vi "LeCroy Wave Series Acquire Waveform.vi"() -> ()   [LabVIEW 2015]
doc: "This example shows how to use autosetup and acquire a waveform on a single channel."
uses:
  Public/Data/Read Single Waveform.vi
  LeCroy Wave Series.lvlib
panel:
  in  "VISA resource name":refnum<visa-resource-name>="VICP::129.175.100.26"
  in  "Reset Scope?":bool
  in  "Perform Auto Setup?":bool
  in  "Source (0: Channel 1)":u16(ring) items=["Channel 1", "Channel 2", "Channel 3", "Channel 4", "Memory 1", "Memory 2", "Memory 3", "Memory 4", "Function 1", "Function 2", "Function 3", "Function 4", "Function 5", "Function 6", "Function 7", "Function 8"]
  in  "Timeout (10000 ms)":u32=10000
  out "Waveform Data":waveform(dbl)(graph)
  # "(c) 2008 - 2012 NATIONAL INSTRUMENTS.  ALL RIGHTS RESERVED."
  # "Directions:\n\n1. Setup the scope to be able to successfully single trigger on a signal applied to the channel selected in the \"Source\" control,  or set Perform Auto Setup? to True to perform an autosetup. \n\n2. On this front panel, enter the VISA Resource name for your scope. (e.g. VICP::123.45.67.8 for TCP/IP, GPIB::5::INSTR for GPIB). Modify the timeout if necessary.\n\n3. For an initial test, set the Reset? and Perform Auto Setup? controls to True, and then run the VI to find the signal.  Leave both set to False for subsequent runs.  The scope's AUX OUT or Cal Out is a good test signal to use."
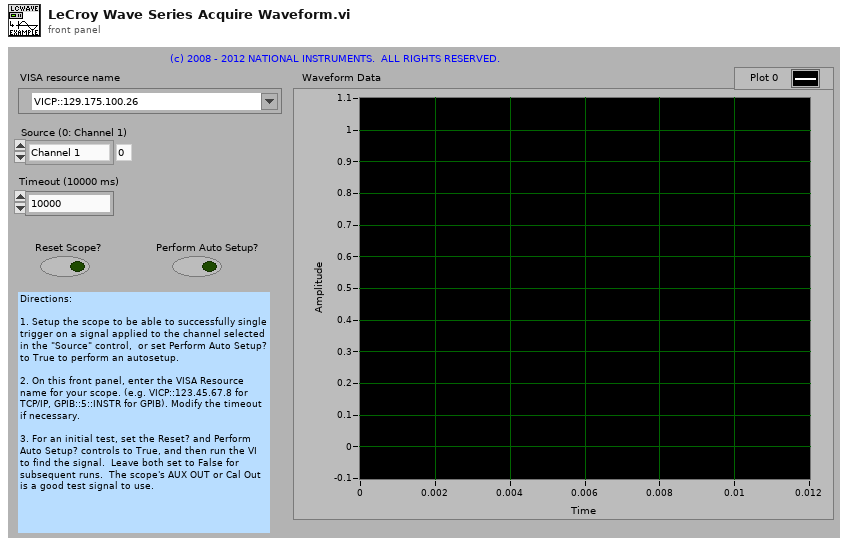
[diagram p1: front panel]
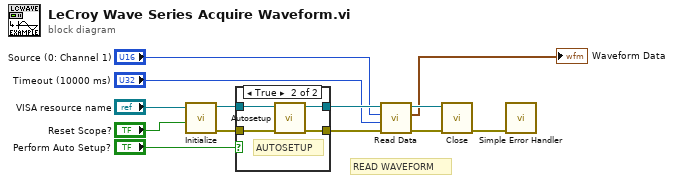
[diagram p0: block diagram]
diagram:
  # "READ WAVEFORM"
  n1 = call "Initialize.vi"("Reset? (T: Yes)"="Reset Scope?", "VISA resource name"="VISA resource name") -> ("error out"=w10:errorcluster, "VISA resource name out"=w9:refnum<visa-resource-name>)  [unwired: 8 in]
  n2 = case shown="True" "Perform Auto Setup?" {
    tunnel: w10 -> [w14 w19]
    tunnel: w9 -> [w15 w18]
    tunnel: [w15 w17] -> w8
    tunnel: [w14 w16] -> w7
    frame False {
    }
    frame True {
      # "AUTOSETUP"
      n3 = call "Autosetup.vi"("error in (no error)"=w19, "VISA resource name"=w18) -> ("error out"=w16:errorcluster, "VISA resource name out"=w17:refnum<visa-resource-name>)  [unwired: 8 in]
    }
  }
  n4 = call-poly "Read Data.vi"("error in (no error)"=w7, "Timeout (10000 ms)"="Timeout (10000 ms)", "Source (0: Channel 1)"="Source (0: Channel 1)", "VISA resource name"=w8) -> ("error out"=w11:errorcluster, "Waveform Data"=→"Waveform Data":waveform(dbl), "VISA resource name out"=w12:refnum<visa-resource-name>)  [unwired: 5 in]
  n5 = call "Close.vi"("error in (no error)"=w11, "VISA resource name"=w12) -> ("error out"=w13:errorcluster)  [unwired: 9 in]
  n6 = call <vilib>:"Simple Error Handler.vi"("error in (no error)"=w13) -> ()  [unwired: 4 in, 5 out]
